vi "3.1.16-Low Pass Steering.vi"(1 "Numeric 2":i32) -> (0 "Numeric":dbl)   [LabVIEW 2010]
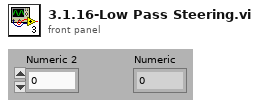
[diagram p1: front panel]
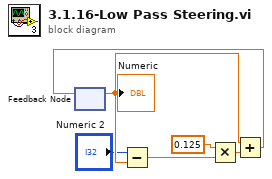
[diagram p0: block diagram]
diagram:
  n1 = feedback #1() -> (w6:dbl)  [unwired: 1 in]
  "Numeric" <- w6
  n2 = Subtract(x="Numeric 2", y=w6) -> (x-y=w2:dbl)
  n3 = Multiply(x=0.125, y=w2) -> (x*y=w4:dbl)
  n4 = Add(x=w6, y=w4) -> (x+y=w5:dbl)
  n5 = feedback-in #1(w5) -> ()
